vi "runscenario not ready.vi"(6 "User Information":T1, 7 "ENV":T3, 8 "error in (no error)":errorcluster, 9 "HTTP Header In (\"\")":string, 10 "Connection Refnum":T2, 11 "http session":T4 {"object data"."time" format="%0.2f"}) -> (0 "error out":errorcluster)   [LabVIEW 2011]
uses:
  server/http/Spartan HTTP Session.ctl
  ITK EXT/http/http_obj.llb/HTTP Session Data.ctl
  ITK EXT/utils/keyedarr.llb/Keyed Array.ctl
  Summitek EXT/ODBC/SQL Controls/Connection Refnum.ctl
  server/database/Users/User Record.ctl
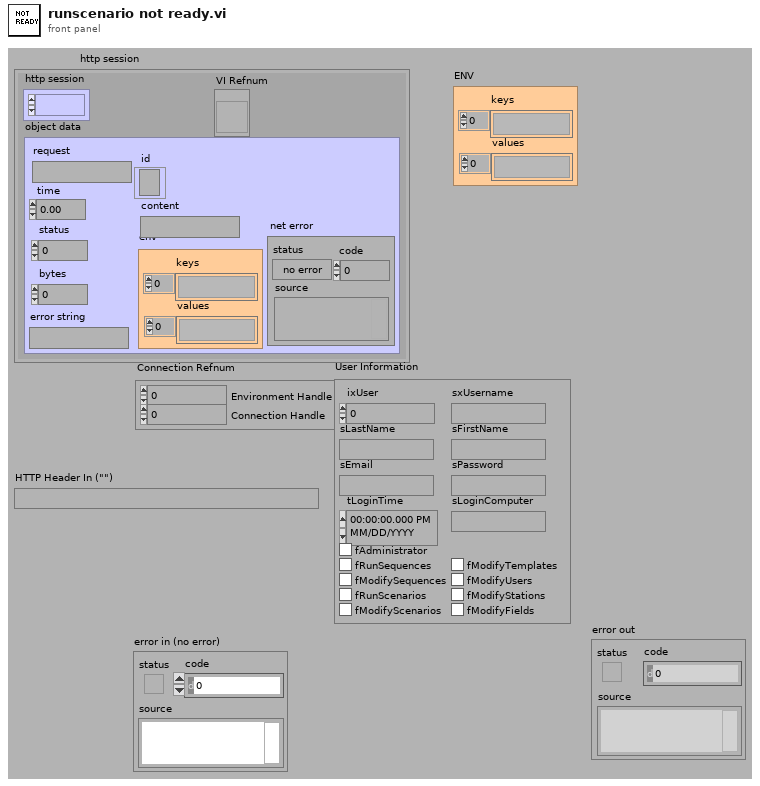
[diagram p1: front panel]
types:
  T1 = typedef "User Record.ctl" = cluster{"ixUser":i32, "sxUsername":string, "sLastName":string, "sFirstName":string, "sEmail":string, "sPassword":string, "tLoginTime":timestamp, "sLoginComputer":string, "fAdministrator":bool, "fRunSequences":bool, "fModifySequences":bool, "fRunScenarios":bool, "fModifyScenarios":bool, "fModifyTemplates":bool, "fModifyUsers":bool, "fModifyStations":bool, "fModifyFields":bool}
  T2 = typedef "Connection Refnum.ctl" = cluster{"Environment Handle":i32, "Connection Handle":i32}
  T3 = typedef "Keyed Array.ctl" = cluster{"keys":string[], "values":string[]}
  T4 = typedef "Spartan HTTP Session.ctl" = cluster{"http session":refnum<k1>, "object data":T5, "VI Refnum":refnum<vi>}
  T5 = typedef "HTTP Session Data.ctl" = cluster{"request":string, "time":dbl, "status":i32, "error string":string, "bytes":i32, "env":T3, "content":string, "id":refnum<k5>, "net error":errorcluster}
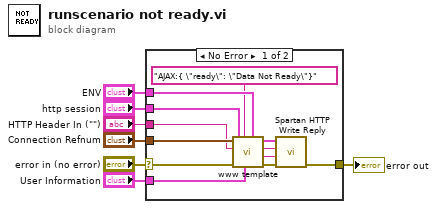
[diagram p0: block diagram]
diagram:
  n1 = case shown="No Error" "error in (no error)" {
    selector: "error in (no error)" -> [w9 w19]
    tunnel: "http session" -> [w16 _]
    tunnel: "ENV" -> [w15 _]
    tunnel: "Connection Refnum" -> [w14 _]
    tunnel: "HTTP Header In (\"\")" -> [w13 _]
    tunnel: "User Information" -> [w12 _]
    tunnel: [w10 w19] -> w2
    frame No Error {
      n2 = call "www template.vi"("ENV"=w15, "User Information"=w12, "Template (\"\")"="AJAX:{ \"ready\": \"Data Not Ready\"}" ("Template (\"\")"), "error in (no error)"=w9, "HTTP Header In (\"\")"=w13, "Connection Refnum"=w14) -> ("error out"=w11:errorcluster, "HTTP Template Content"=w18:string, "HTTP Header Out"=w17:string)  [unwired: 1 in, 2 out]
      n3 = call "Spartan HTTP Write Reply.vi"("error in (no error)"=w11, "content"=w18, "header"=w17, "http session"=w16) -> ("error out"=w10:errorcluster)  [unwired: 1 in, 6 out]
    }
    frame Error {
    }
  }
  "error out" <- w2
